vi "New Topic.vi"(9 "New Topic Data":variant, 10 "Name":string, 11 "Use Type Input As Initial Value?":bool) -> (0 "error out":errorcluster, 3 "Topic out":refnum<class "Topic.lvclass">)   [LabVIEW 2015, in "Mediator.lvlib" / "Topic.lvclass"]
doc: "<License>\nCopyright © 2017 Composed Systems, LLC | All rights reserved\nwww.composed.io\n\nAuthor: Ethan Stern <ethan.stern@composed.io>\n\nThis software is provided \"AS IS\" WITHOUT WARRANTIES, either express or implied, AND IS FOR EDUCATIONAL PURPOSES ONLY.\n</License>"
uses:
  Topic.lvclass
  Topic.lvclass/Topic.ctl
  <vilib>/Composed Systems/Variant Extensions/VariantExtensions.lvlib
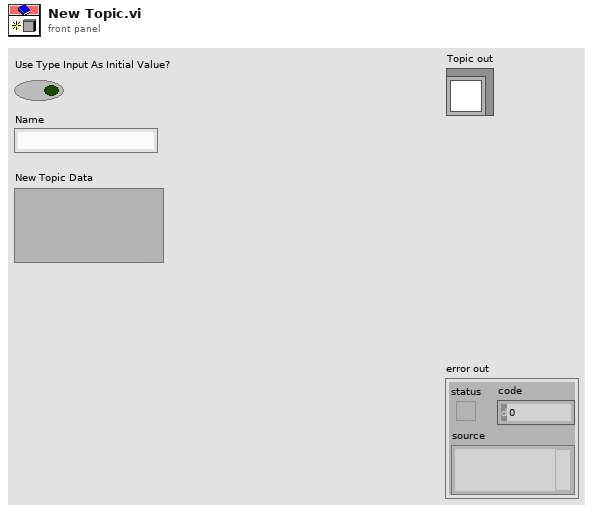
[diagram p1: front panel]
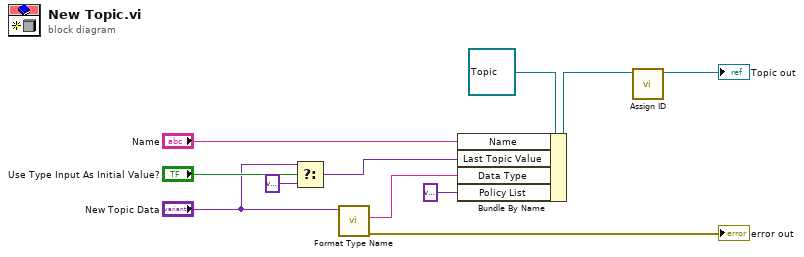
[diagram p0: block diagram]
diagram:
  n1 = Select(t="New Topic Data", s="Use Type Input As Initial Value?", f=variant) -> (s? t:f=w2:variant)
  n2 = call <vilib>:"Format Type Name.vi"("Data Type"="New Topic Data") -> ("error out"=→"error out":errorcluster, "Type Name"=w7:string)  [unwired: 9 in]
  n3 = Bundle By Name(cluster=refnum<class "Topic.lvclass"> refnum ("Topic in"), "Name"="Name", "Last Topic Value"=w2, "Data Type"=w7, "Policy List"=variant ("Subscriber List")) -> (w10:refnum<class "Topic.lvclass">)
  n4 = call "Assign ID.vi"("Topic in"=w10) -> ("Topic out"=→"Topic out":refnum<class "Topic.lvclass">)  [unwired: 10 in]
